vi "Get Case Matching.vi"(1 "string matching":T1=enum."system") -> (0 "match case":bool)   [LabVIEW 2015, in "TLB` Template.lvlib" / "Tools_String.lvlib"]
doc: "TLB Prime - Application Template 1.3.0.24\nNorm Kirchner, NI Systems Engineering - NI\nCopyright (c) 2014, NI"
uses:
  Tools_String.lvlib
  <vilib>/FTP/util/Case Matching.ctl
  <vilib>/FTP/NI_FTP.lvlib
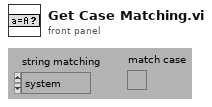
[diagram p1: front panel]
types:
  T1 = typedef "NI_FTP.lvlib/Case Matching.ctl" = enum16{"a != A", "a == A", "system"}
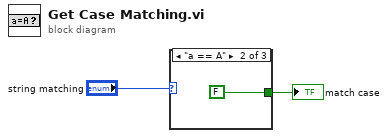
[diagram p0: block diagram]
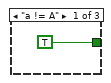
[diagram p2: hidden frame]
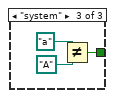
[diagram p3: hidden frame]
diagram:
  n1 = case shown="\"a == A\"" "string matching" {
    tunnel: [TRUE FALSE w5] -> w1
    frame "a != A" {
    }
    frame "a == A" {
    }
    frame "system" {
      n2 = Not Equal?(x=path "a", y=path "A") -> (x != y?=w5:bool)
    }
  }
  "match case" <- w1
